vi "determine_offset_and_factor_for_saving.vi"(8 "error in (no error)":errorcluster, 11 "DataCollectionMG091001IntrinsicImaging in":refnum<class "DataCollectionMG091001IntrinsicImaging.lvclass">) -> (0 "error out":errorcluster, 1 "factor":dbl, 2 "offset":dbl, 3 "DataCollectionMG091001IntrinsicImaging out":refnum<class "DataCollectionMG091001IntrinsicImaging.lvclass">)   [LabVIEW 2010, in "DataCollectionMG091001IntrinsicImaging.lvclass"]
uses:
  DataCollectionMG091001IntrinsicImaging.lvclass
  DataCollectionMG091001IntrinsicImaging.lvclass/DataCollectionMG091001IntrinsicImaging.ctl
  common/classes/ImageCollection/ImageCollection/ImageCollection.lvclass
panel:
  in  "max supported in target file":dbl=65535.0
  in  "min supported in target file":dbl
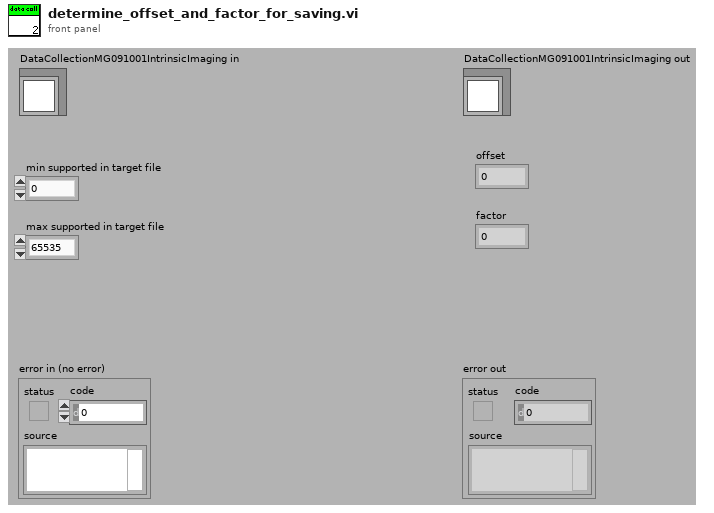
[diagram p1: front panel]
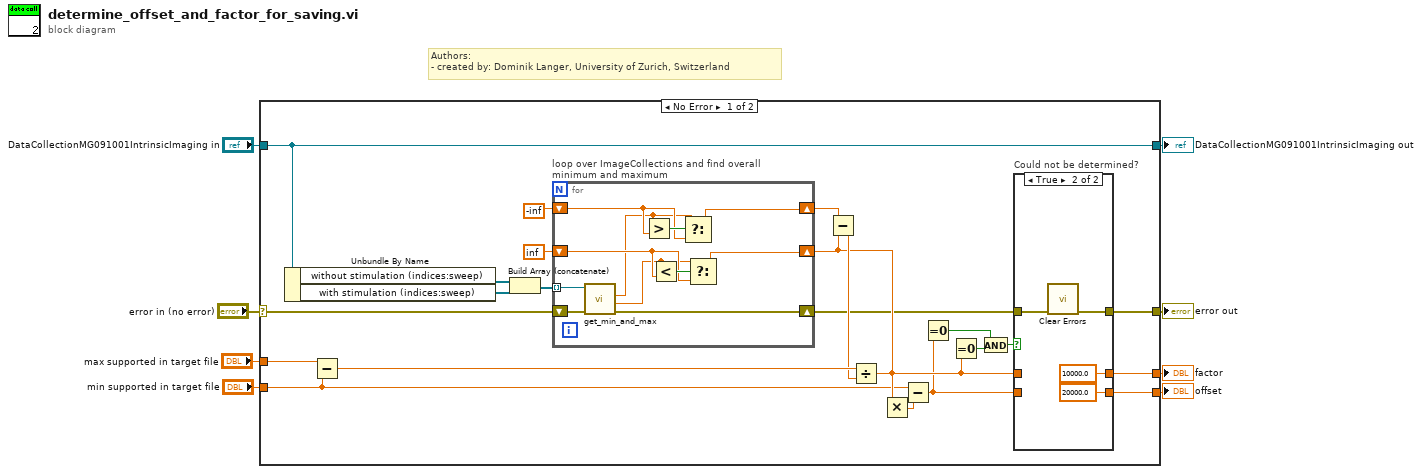
[diagram p0: block diagram]
diagram:
  # "Authors: \n- created by: Dominik Langer, University of Zurich, Switzerland"
  n1 = case shown="No Error" "error in (no error)" {
    selector: "error in (no error)" -> [w28 w51]
    tunnel: [w10 w51] -> w7
    tunnel: [w31 w50] -> w5
    tunnel: "DataCollectionMG091001IntrinsicImaging in" -> [w31 w50]
    tunnel: "max supported in target file" -> [w20 _]
    tunnel: "min supported in target file" -> [w19 _]
    tunnel: [w12 _] -> w2
    tunnel: [w11 _] -> w1
    frame No Error {
      n2 = Unbundle By Name(w31) -> ("without stimulation (indices:sweep)"=w29:refnum<class "ImageCollection.lvclass">[], "with stimulation (indices:sweep)"=w30:refnum<class "ImageCollection.lvclass">[])
      n3 = Subtract(x=w20, y=w19) -> (x-y=w25:dbl)
      n4 = Build Array (concatenate)(w29, w30) -> (w27:refnum<class "ImageCollection.lvclass">[])
      n5 = for "loop over ImageCollections and find overall minimum and maximum" {
        shift-right: [w42] -> w15
        shift-left: w28 -> [w43]
        shift-right: [w48] -> w26
        shift-left: -inf -> [w47]
        shift-right: [w44] -> w23
        shift-left: inf -> [w45]
        tunnel: w27 -> [w41] mode=indexing
        n6 = call "get_min_and_max.vi"("error in (no error)"=w43, "ImageCollection in"=w41) -> ("error out"=w42:errorcluster, "minimum"=w40:dbl, "maximum"=w39:dbl)  [unwired: 5 in, 2 out]
        n7 = Greater?(x=w39, y=w47) -> (0:w49:bool)
        n8 = Less?(x=w40, y=w45) -> (x < y?=w46:bool)
        n9 = Select(t=w39, s=w49, f=w47) -> (s? t:f=w48:dbl)
        n10 = Select(t=w40, s=w46, f=w45) -> (s? t:f=w44:dbl)
      }
      n11 = Subtract(x=w26, y=w23) -> (x-y=w24:dbl)
      n12 = Divide(x=w25, y=w24) -> (x/y=w14:dbl)
      n13 = Multiply(x=w23, y=w14) -> (x*y=w18:dbl)
      n14 = Subtract(x=w19, y=w18) -> (x-y=w13:dbl)
      n15 = Equal To 0?(x=w13) -> (x = 0?=w17:bool)
      n16 = Equal To 0?(x=w14) -> (x = 0?=w16:bool)
      n17 = And(x=w17, y=w16) -> (x .and. y?=w9:bool)
      n18 = case "Could not be determined?" shown="True" w9 {
        tunnel: w15 -> [w32 w38]
        tunnel: w14 -> [w34 _]
        tunnel: w13 -> [w33 _]
        tunnel: [w34 10000.0] -> w12
        tunnel: [w33 20000.0] -> w11
        tunnel: [w32 w35] -> w10
        frame False {
        }
        frame True {
          n19 = call <vilib>:"Clear Errors.vi"("error in (no error)"=w38) -> ("error out"=w35:errorcluster)  [unwired: 6 in]
        }
      }
    }
    frame Error {
    }
  }
  "error out" <- w7
  "DataCollectionMG091001IntrinsicImaging out" <- w5
  "factor" <- w2
  "offset" <- w1
